vi "Module Timeout--constant.vi"() -> (3 "Module Timeout":i32)   [LabVIEW 2022 SP3, in "GenNet-Server.lvlib"]
doc: "A module-wide common value to use as the timeout for various synchronization actions.\n____\nHAMPEL SOFTWARE ENGINEERING v3.8.0 (2023-12-18 14:41)"
uses:
  GenNet-Server.lvlib
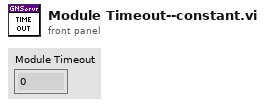
[diagram p1: front panel]
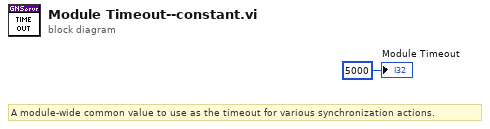
[diagram p0: block diagram]
diagram:
  # "A module-wide common value to use as the timeout for various synchronization actions."
  "Module Timeout" <- 5000 ("Module Timeout")
